vi "add StrainCell initialize.vi"(9 "字符串":string) -> (1 "连接的字符串":string, 3 "ok or cancel":bool=TRUE)   [LabVIEW 2019, in "nematic.lvlib" / "Copy of StrainCell.lvlib"]
uses:
  nematic/Copy of StrainCell.lvlib
  lib/Keithley 622x/Configure/Delta PDelta DCon Modes/Typedefs/KE622x -- Delta Mode Params.ctl
  lib/Keithley 622x/Configure/Delta PDelta DCon Modes/Low Level/Typedefs/KE622x -- Delta PDelta Mode High Level.ctl
  lib/Keithley 622x/Configure/Delta PDelta DCon Modes/Low Level/Typedefs/KE622x -- Delta PDelta Mode Low Level.ctl
  lib/Keithley 622x/Configure/Delta PDelta DCon Modes/Low Level/Typedefs/KE622x -- Delta DCon Mode Delay.ctl
  lib/Keithley 622x/Configure/Delta PDelta DCon Modes/Low Level/Typedefs/KE622x -- Delta PDelta Mode Num Cycles Mode.ctl
  lib/Keithley 622x/Configure/Delta PDelta DCon Modes/Low Level/Typedefs/KE622x -- Delta PDelta Mode Num Cycles.ctl
  lib/Keithley 622x/Configure/2182 -A/Low Level/Typedefs/KE2182 -- Voltage Ranges.ctl
  lib/Keithley 622x/Configure/2182 -A/Low Level/Typedefs/KE2182 -- Filter Type.ctl
  lib/Keithley 622x/Configure/2182 -A/Low Level/Typedefs/KE2182 -- Filter Count.ctl
  lib/Keithley 622x/Configure/2182 -A/Low Level/Typedefs/KE2182 -- Filter Window.ctl
  lib/Keithley 622x/Configure/2182 -A/Low Level/Typedefs/KE2182 -- NPLCs.ctl
  lib/Keithley 622x/Configure/Source/Typedefs/KE622x -- Voltage Limit.ctl
  lib/Keithley 622x/Keithley 622x.lvlib
panel:
  in  "RP100 Reset ?(True)":bool
  in  "Voltage Limit (V)":T1=10.0 min=0.1 max=105.0 step=0.01 format="%.2p"
  in  "2812 -A Params In":T7={"Auto Range?"=FALSE, "Man / Selected\nRange"=enum."10mV", "Enable Digital\nFilter?"=FALSE, "Filter Type"=enum."Moving", "Filter Count"=10, "Filter\nWindow (%)"=0.01, "Enable Analog\nFilter?"=FALSE, "NPLCs"=5} {"Filter\nWindow (%)" min=0.0 max=10.0 step=0.01 format="%.2f"; "Filter Count" min=1 max=100; "NPLCs" min=1 max=10}
  in  "Delta Mode Params In":T8={"High Level (A)"=0.001, "Low Level (A)"=-0.001, "Delay (s)"=0.02, "Num Cycles Mode"=enum."Finite Count", "Finite Count"=6, "Abort On\nCompliance?"=FALSE, "Cold Swithing\nMode Enabled?"=FALSE} {"Finite Count" min=1 max=65536; "Low Level (A)" min=-0.105 max=0.0 format="%.3p"; "High Level (A)" min=0.0 max=0.105 format="%.3p"; "Delay (s)" min=0.001 max=9999.999 format="%.3f"}
  out "error out":errorcluster
  in  "load":bool
  in  "cancel":bool
  in  "ok":bool
  out "错误输出":errorcluster
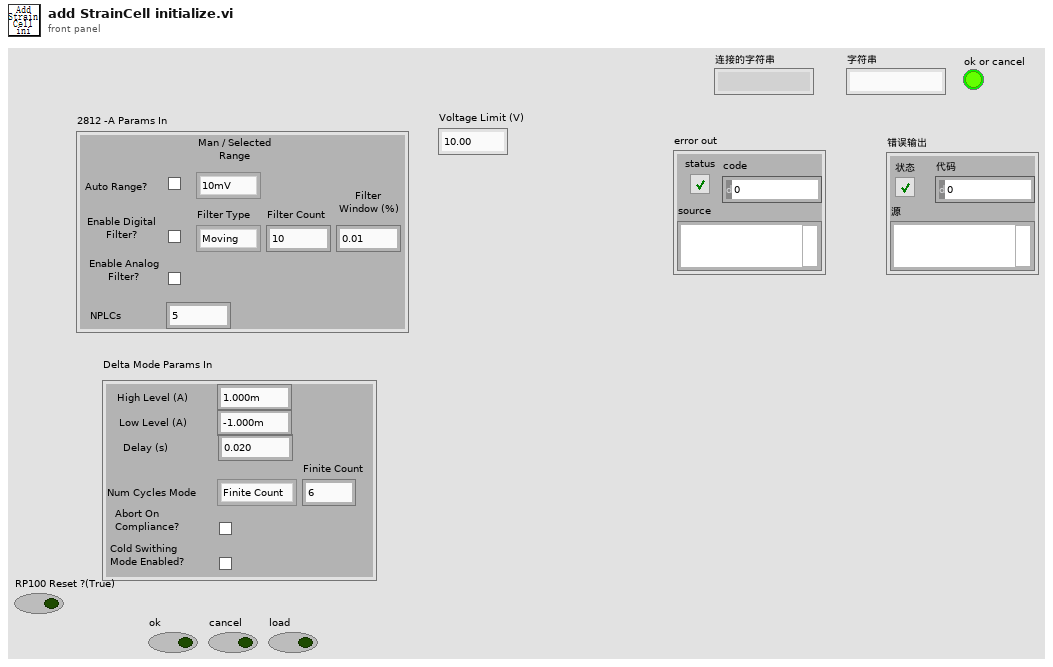
[diagram p1: front panel]
types:
  T1 = typedef "Keithley 622x.lvlib/KE622x -- Voltage Limit.ctl" = dbl
  T2 = typedef "Keithley 622x.lvlib/KE2182 -- Voltage Ranges.ctl" = enum16{"10mV", "100mV", "1V", "10V", "100V"}
  T3 = typedef "Keithley 622x.lvlib/KE2182 -- Filter Type.ctl" = enum16{"Moving", "Repeat"}
  T4 = typedef "Keithley 622x.lvlib/KE2182 -- Filter Count.ctl" = u32
  T5 = typedef "Keithley 622x.lvlib/KE2182 -- Filter Window.ctl" = dbl
  T6 = typedef "Keithley 622x.lvlib/KE2182 -- NPLCs.ctl" = u32
  T7 = cluster{"Auto Range?":bool, "Man / Selected\nRange":T2, "Enable Digital\nFilter?":bool, "Filter Type":T3, "Filter Count":T4, "Filter\nWindow (%)":T5, "Enable Analog\nFilter?":bool, "NPLCs":T6}
  T8 = typedef "Keithley 622x.lvlib/KE622x -- Delta Mode Params.ctl" = cluster{"High Level (A)":T9, "Low Level (A)":T10, "Delay (s)":T11, "Num Cycles Mode":T12, "Finite Count":T13, "Abort On\nCompliance?":bool, "Cold Swithing\nMode Enabled?":bool}
  T9 = typedef "Keithley 622x.lvlib/KE622x -- Delta PDelta Mode High Level.ctl" = dbl
  T10 = typedef "Keithley 622x.lvlib/KE622x -- Delta PDelta Mode Low Level.ctl" = dbl
  T11 = typedef "Keithley 622x.lvlib/KE622x -- Delta DCon Mode Delay.ctl" = dbl
  T12 = typedef "Keithley 622x.lvlib/KE622x -- Delta PDelta Mode Num Cycles Mode.ctl" = enum16{"Finite Count", "Infinite"}
  T13 = typedef "Keithley 622x.lvlib/KE622x -- Delta PDelta Mode Num Cycles.ctl" = u32
  T14 = enum16{"open", "replace", "create", "open or create", "replace or create"}
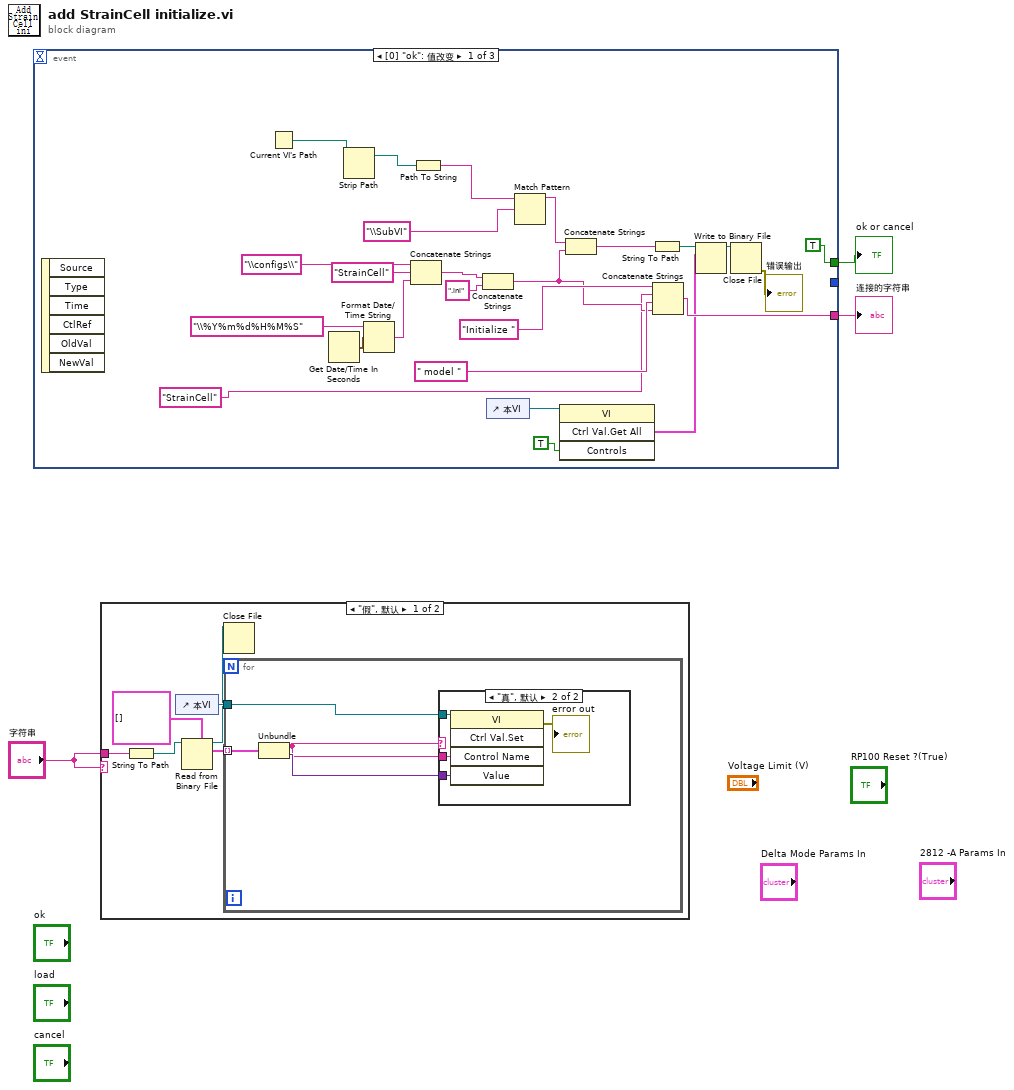
[diagram p0: block diagram]
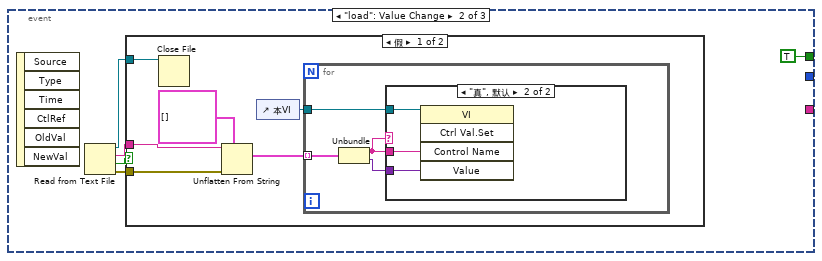
[diagram p4: hidden frame]
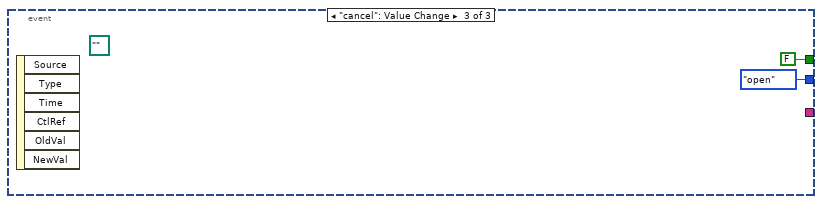
[diagram p7: hidden frame]
diagram:
  n1 = event shown="[0] \"ok\": 值改变" {
    selector: _ -> [_ _ _]
    dyn-events: _ -> [_ _ _]
    timeout: _ -> [_ _ _]
    tunnel: [_ _ T14."open" ("operation(0:open)")] -> _
    tunnel: [TRUE TRUE FALSE] -> w3
    tunnel: [w21 _ _] -> w1
    event "ok": Value Change {
      n2 = event-data() -> ()  [unwired: 1 in, 6 out]
      n3 = Current VI's Path() -> (path=w12:path)
      n4 = Get Date/Time In Seconds() -> (seconds since 1Jan1904=w14:timestamp)
      n5 = Strip Path(path=w12) -> (stripped path=w17:path)  [unwired: 1 out]
      n6 = Format Date/Time String(time format string (%c)="\\%Y%m%d%H%M%S", seconds (now)=w14) -> (date/time string=w13:string)  [unwired: 1 in]
      n7 = Concatenate Strings("\\configs\\" ("字符串"), "StrainCell" ("字符串"), w13) -> (w9:string)
      n8 = Path To String(path=w17) -> (string=w11:string)
      n9 = Concatenate Strings(w9, ".ini" ("字符串")) -> (w6:string)
      n10 = control-ref of="本VI"() -> (w27:refnum<vi>)
      n11 = Match Pattern(string=w11, regular expression="\\SubVI" ("正则表达式")) -> (before substring=w7:string)  [unwired: 1 in, 3 out]
      n12 = invoke class="VI" method="Ctrl Val.Get All"(reference=w27, "Controls"=TRUE ("控件")) -> ("Get All Control Values Variant"=w19:cluster{"Name":string, "Variant Data":variant}[])  [unwired: 2 in, 3 out]
      n13 = Concatenate Strings(w7, w6) -> (w5:string)
      n14 = String To Path(string=w5) -> (path=w20:path)
      n15 = Concatenate Strings("Initialize " ("字符串"), "StrainCell" ("字符串"), " model " ("字符串"), w6) -> (w21:string)
      n16 = Write to Binary File(file (use dialog)=w20, data=w19) -> (refnum out=w18:refnum<file>)  [unwired: 4 in, 2 out]
      n17 = Close File(refnum=w18) -> (error out=→"错误输出":errorcluster)  [unwired: 1 in, 1 out]
    }
    event "load": Value Change {
      n18 = event-data() -> ()  [unwired: 1 in, 6 out]
      n19 = Read from Text File() -> (refnum out=w32:refnum<file>, text=w30:string, cancelled=w29:bool, error out=w31:errorcluster)  [unwired: 4 in]
      n20 = case shown="假" w29 {
        tunnel: w32 -> [w39 _]
        tunnel: w31 -> [w37 _]
        tunnel: w30 -> [w36 _]
        frame False {
          n21 = Close File(refnum=w39) -> ()  [unwired: 1 in, 2 out]
          n22 = Unflatten From String(type=cluster{"Name":string, "Variant Data":variant}[] [] ("控件值:获取全部"), binary string=w36, error in (no error)=w37) -> (value=w35:cluster{"Name":string, "Variant Data":variant}[])  [unwired: 2 in, 2 out]
          n23 = control-ref of="本VI"() -> (w34:refnum<vi>)
          n24 = for {
            tunnel: w35 -> [w43] mode=indexing
            tunnel: w34 -> [w42]
            n25 = Unbundle(w43) -> ("Name"=w40:string, "Variant Data"=w41:variant)
            n26 = case shown="\"真\", 默认" w40 {
              tunnel: w42 -> [_ w46]
              tunnel: w40 -> [_ w45]
              tunnel: w41 -> [_ w44]
              frame "cancel", "load", "ok" {
              }
              frame "真", Default {
                n27 = invoke class="VI" method="Ctrl Val.Set"(reference=w46, "Control Name"=w45, "Value"=w44) -> ()  [unwired: 2 in, 5 out]
              }
            }
          }
        }
        frame True {
        }
      }
    }
    event "cancel": Value Change {
      (unwired) path "" ("path")
      n28 = event-data() -> ()  [unwired: 1 in, 6 out]
    }
  }
  "ok or cancel" <- w3
  "连接的字符串" <- w1
  n29 = case shown="\"假\", 默认" "字符串" {
    tunnel: "字符串" -> [w54 _]
    frame "假", Default {
      n30 = String To Path(string=w54) -> (path=w52:path)
      n31 = control-ref of="本VI"() -> (w53:refnum<vi>)
      n32 = Read from Binary File(5:cluster{"Name":string, "Variant Data":variant}[] [] ("控件值:获取全部"), 11:w52) -> (2:w50:cluster{"Name":string, "Variant Data":variant}[], 3:w49:refnum<file>)  [unwired: 4 in, 2 out]
      n33 = Close File(refnum=w49) -> ()  [unwired: 1 in, 2 out]
      n34 = for {
        tunnel: w50 -> [w58] mode=indexing
        tunnel: w53 -> [w57]
        n35 = Unbundle(w58) -> ("Name"=w55:string, "Variant Data"=w56:variant)
        n36 = case shown="\"真\", 默认" w55 {
          tunnel: w57 -> [_ w62]
          tunnel: w55 -> [_ w61]
          tunnel: w56 -> [_ w60]
          frame "cancel", "load", "ok" {
          }
          frame "真", Default {
            n37 = invoke class="VI" method="Ctrl Val.Set"(reference=w62, "Control Name"=w61, "Value"=w60) -> (error out=→"error out":errorcluster)  [unwired: 2 in, 4 out]
          }
        }
      }
    }
    frame "" {
    }
  }
